vi "test Parse Clusters.vi"(8 "error in (no error)":errorcluster, 11 "TestCase in":refnum<class "Parse Bitfile Test Case.lvclass">) -> (0 "error out":errorcluster, 3 "TestCase out":refnum<class "Parse Bitfile Test Case.lvclass">)   [LabVIEW 2015]
uses:
  Parse Bitfile Test Case.lvclass
  <userlib>/_OpenG.lib/file/file.llb/Append Path to Root if Relative - Scalar__ogtk.vi
  <vilib>/addons/_JKI Toolkits/VI Tester/TestCase.llb/TestCase.lvclass
  System Explorer/Engine Simulation Toolkit System Explorer.lvlib
panel:
  out "EPS IP LUT":variant
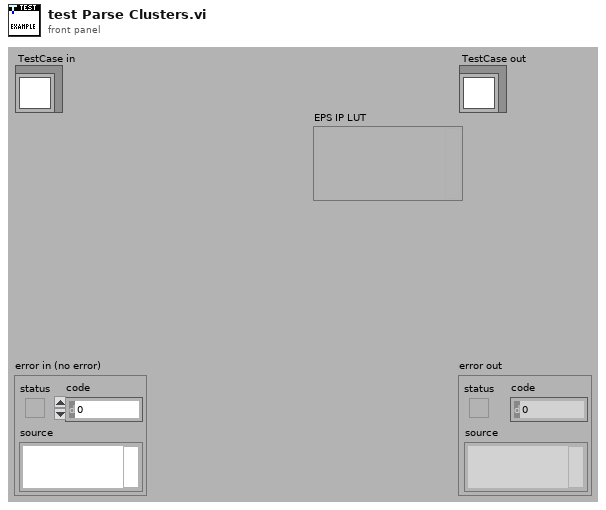
[diagram p1: front panel]
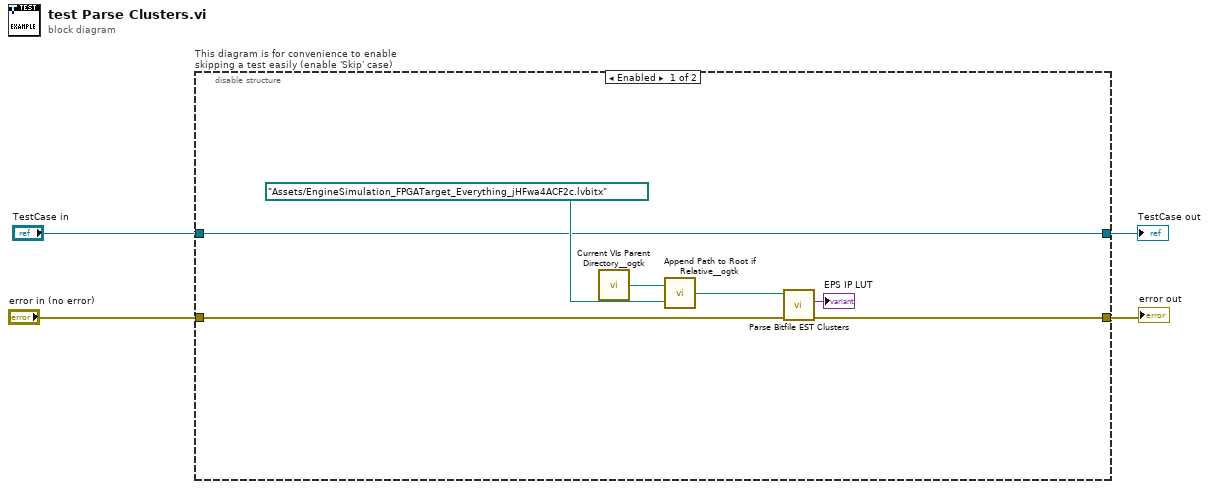
[diagram p0: block diagram]
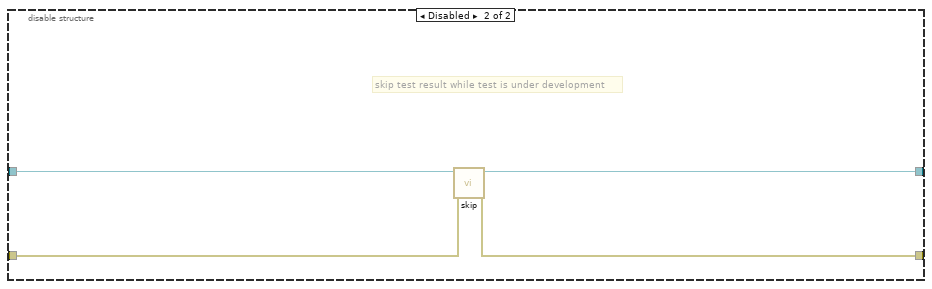
[diagram p2: hidden frame]
diagram:
  n1 = disable-structure "This diagram is for convenience to enable skipping a test easily (enable 'Skip' case)" shown="Enabled" {
    disable-tunnel: "TestCase in" -> [w9 w15]
    disable-tunnel: [w9 w13] -> w1
    disable-tunnel: [w6 w14] -> w3
    disable-tunnel: "error in (no error)" -> [w7 w12]
    frame Enabled {
      n2 = call <userlib>:"Current VIs Parent Directory__ogtk.vi"() -> ("Parent Directory (+ Relative)"=w11:path)  [unwired: 5 in]
      n3 = call-poly <userlib>:"Append Path to Root if Relative__ogtk.vi"("Absolute or Relative Path"=path "Assets/EngineSimulation_FPGATarget_Everything_jHFwa4ACF2c.lvbitx" ("bitfile path"), "Root Path"=w11) -> ("Absolute or Appended Path"=w8:path)
      n4 = call "Parse Bitfile EST Clusters.vi"("error in (no error)"=w7, "bitfile path"=w8) -> ("error out"=w6:errorcluster, "EPS IP LUT"=→"EPS IP LUT":variant)  [unwired: 5 in, 3 out]
    }
    frame Disabled {
      # "skip test result while test is under development"
      n5 = call <vilib>:"skip.vi"("error in (no error)"=w12, "TestCase in"=w15) -> ("error out"=w14:errorcluster, "TestCase out"=w13:refnum<class "Parse Bitfile Test Case.lvclass">)  [unwired: 8 in]
    }
  }
  "error out" <- w3
  "TestCase out" <- w1
